vi "JSONEscapeString.vi"(8 "error in (no error)":errorcluster, 11 "raw":string) -> (0 "error out":errorcluster, 3 "escaped":string)   [LabVIEW 2026, in "Lumberjack.lvlib"]
doc: "Escapes a string into a JSON string literal: backslash and double-quote, the named control chars (\\n \\r \\t \\b \\f), any other U+0000–U+001F as \\u00xx, then wraps in double quotes. Pure, no dependencies. Used by JSONLayout.Format for every emitted value."
uses:
  Lumberjack.lvlib
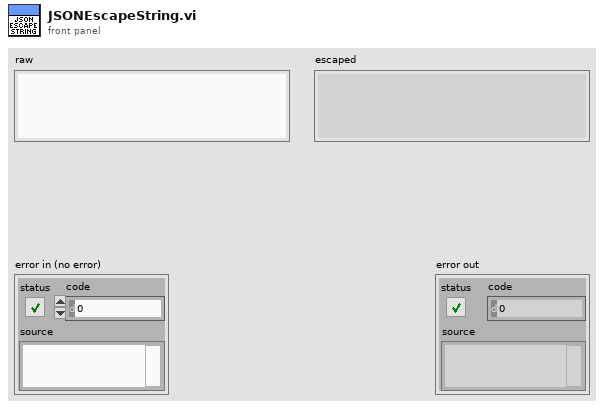
[diagram p1: front panel]
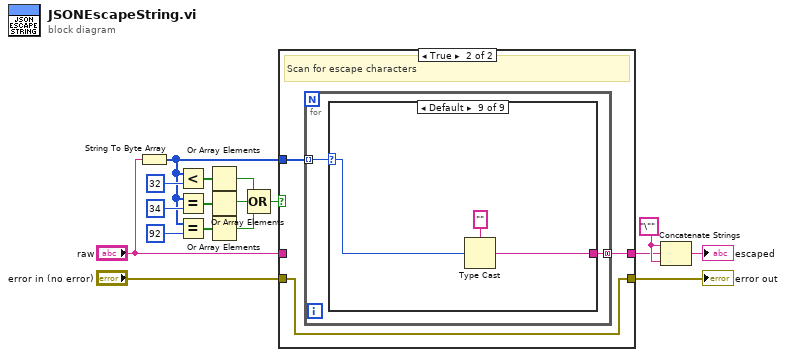
[diagram p0: block diagram]
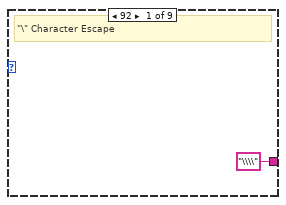
[diagram p3: hidden frame]
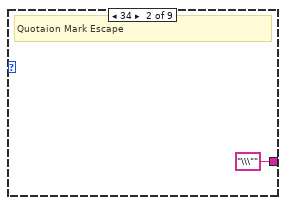
[diagram p4: hidden frame]
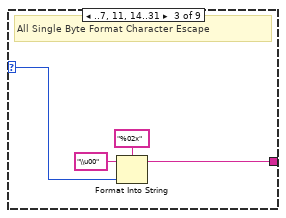
[diagram p5: hidden frame]
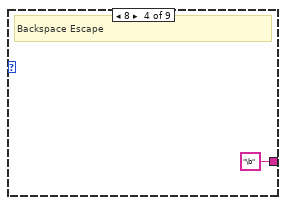
[diagram p6: hidden frame]
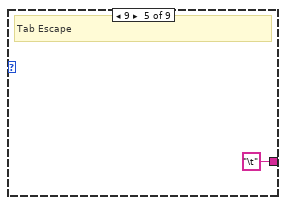
[diagram p7: hidden frame]
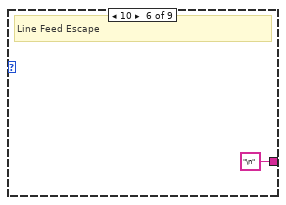
[diagram p8: hidden frame]
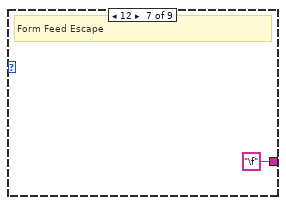
[diagram p9: hidden frame]
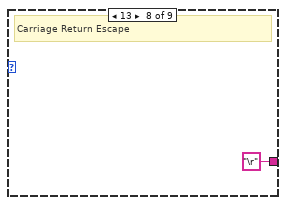
[diagram p10: hidden frame]
diagram:
  w3 = "\"" ("string")
  n1 = String To Byte Array(string="raw") -> (unsigned byte array=w14:u8[])
  n2 = Less?(x=w14, y=u8 32) -> (x < y?=w12:bool[])
  n3 = Equal?(x=w14, y=u8 34) -> (x = y?=w11:bool[])
  n4 = Equal?(x=w14, y=u8 92) -> (x = y?=w10:bool[])
  n5 = Or Array Elements(Boolean array=w12) -> (logical OR=w9:bool)
  n6 = Or Array Elements(Boolean array=w11) -> (logical OR=w8:bool)
  n7 = Or Array Elements(Boolean array=w10) -> (logical OR=w7:bool)
  n8 = Compound Arithmetic op=OR(w9, w8, w7) -> (w6:bool)
  n9 = case shown="True" w6 {
    tunnel: "error in (no error)" -> [w19 w20]
    tunnel: w14 -> [_ w22]
    tunnel: "raw" -> [w18 _]
    tunnel: [w19 w20] -> w4
    tunnel: [w18 w21] -> w2
    frame False {
      # "Nothing to Escape"
    }
    frame True {
      # "Scan for escape characters"
      n10 = for {
        tunnel: w22 -> [w24] mode=indexing
        tunnel: [w23] -> w21 mode=concatenating
        n11 = case shown="Default" w24 {
          selector: w24 -> [_ _ w30 _ _ _ _ _ w38]
          tunnel: ["\\\\" "\\\"" w28 "\b" "\t" "\n" "\f" "\r" w37] -> w23
          frame 92 {
            # "\"\\\" Character Escape"
          }
          frame 34 {
            # "Quotaion Mark Escape"
          }
          frame ..7, 11, 14..31 {
            # "All Single Byte Format Character Escape"
            n12 = Format Into String(format string="%02x", initial string="\\u00", w30) -> (resulting string=w28:string)  [unwired: 1 in, 1 out]
          }
          frame 8 {
            # "Backspace Escape"
          }
          frame 9 {
            # "Tab Escape"
          }
          frame 10 {
            # "Line Feed Escape"
          }
          frame 12 {
            # "Form Feed Escape"
          }
          frame 13 {
            # "Carriage Return Escape"
          }
          frame Default {
            n13 = Type Cast(type="", x=w38) -> (*(type *) &x=w37:string)
          }
        }
      }
    }
  }
  "error out" <- w4
  n14 = Concatenate Strings(w3, w2, w3) -> (→"escaped":string)
